vi "RVC Sensor.vi"(1 "x2":dbl=0.1 format="%#_13g", 2 "Pose":dbl[](array[numeric]), 4 "Light Sense X position":dbl=60.0, 5 "y2":dbl format="%#_13g", 8 "Light Sense Y position":dbl=90.0) -> (7 "sensor":dbl)   [LabVIEW 2014]
uses:
  <vilib>/Analysis/baseanly.llb/Real A x B.vi
  <vilib>/Analysis/NI_AALBase.lvlib
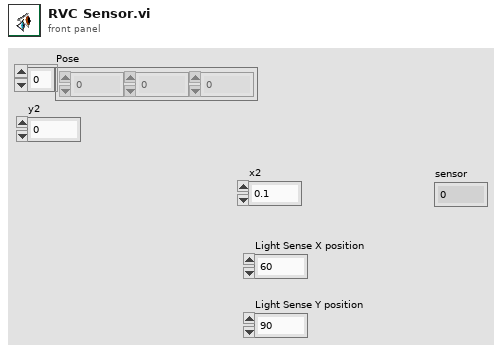
[diagram p1: front panel]
types:
  T1 = typedef "NI_Matrix.lvlib/RealMatrix.ctl" = dbl[][]
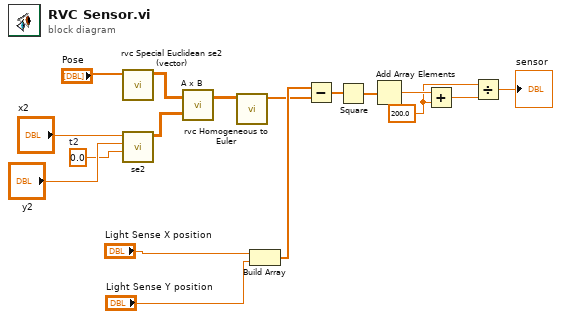
[diagram p0: block diagram]
diagram:
  w4 = 0.0  # t2
  w11 = 200.0 ("y")
  n1 = call "rvc Special Euclidean se2 (vector).vi"("Pose"="Pose") -> ("T"=w7:dbl[][])  [unwired: 9 in, 1 out]
  n2 = call "se2.vi"("theta"=w4, "y"="y2", "x"="x2") -> ("T"=w1:dbl[][])  [unwired: 7 in, 1 out]
  n3 = call-poly <vilib>:"A x B.vi"("B"=w1, "A"=w7) -> ("A x B"=w3:T1)  [unwired: 1 out]
  n4 = call "rvc Homogeneous to Euler.vi"("T"=w3) -> ("Array"=w2:dbl[])  [unwired: 6 in, 4 out]
  n5 = Build Array("Light Sense X position", "Light Sense Y position") -> (w14:dbl[])
  n6 = Subtract(x=w14, y=w2) -> (x-y=w13:dbl[])
  n7 = Square(x=w13) -> (x^2=w17:dbl[])
  n8 = Add Array Elements(numeric array=w17) -> (sum=w12:dbl)
  n9 = Add(x=w12, y=w11) -> (x+y=w10:dbl)
  n10 = Divide(x=w11, y=w10) -> (x/y=→"sensor":dbl)
